vi "Tag_Buffer_Dbl_Input_VIG.vi"(7 "Operation":enum16{"get data", "set data", "initialize"}(ring)=enum."set data", 8 "error in":errorcluster, 9 "Number of Sensors":i32, 11 "tag_data_in":dbl[](array[numeric])) -> (0 "error out":errorcluster, 3 "tag_data_out":dbl[](array[numeric]))   [LabVIEW 2018]
panel:
  # "----TestData Rows---------\n6 -->Flow Rate-(Flow)\n7--->Actual mA (Acutal_Current)\n8-->Temperature (Temp)\n9-->DAQ Sensor 1-Supply Pressure (Supply_Pressure)\n10-->DAQ Sensor 2 - Diff Pressure (50 psid)--(Diff_Pressure_50)\n11-->DAQ Sensor 3 - Back Pressure (output)--(Back_Pressure)\n12-->DAQ Sensor 4- Bypass Pressure--(Bypass_Pressure)\n13-->DAQ Sensor 5 - Diff Pressure (100 psid)--(Diff_Pressure_10)\n14-->DAQ Sensor 6- Unused-(Unused)\n15-->Flow Rate (Raw)--(Flow_Raw)\n16-->Calibrated Flow--(Flow_Cal)\n17-->SG Calibrated --(SG_Cal)"
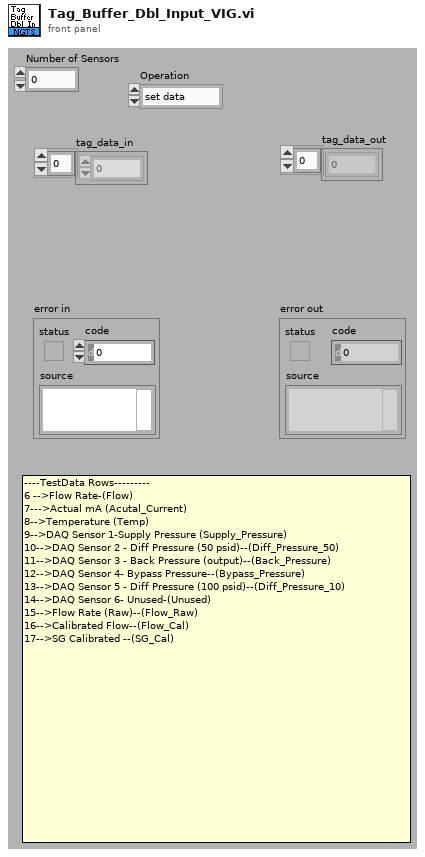
[diagram p1: front panel]
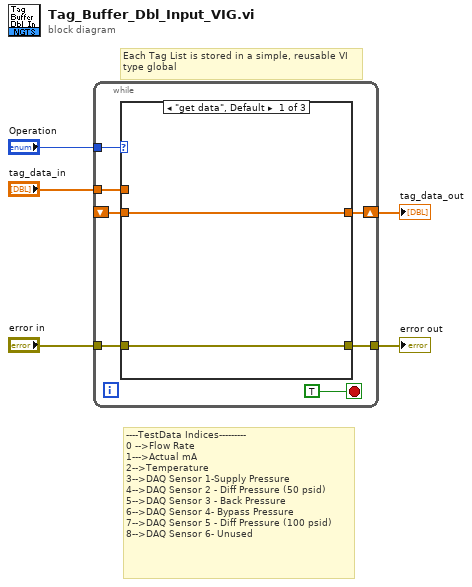
[diagram p0: block diagram]
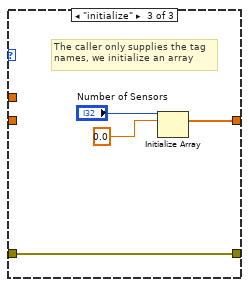
[diagram p3: hidden frame]
diagram:
  # "----TestData Indices---------\n0 -->Flow Rate\n1--->Actual mA \n2-->Temperature\n3-->DAQ Sensor 1-Supply Pressure\n4-->DAQ Sensor 2 - Diff Pressure (50 psid)\n5-->DAQ Sensor 3 - Back Pressure\n6-->DAQ Sensor 4- Bypass Pressure\n7-->DAQ Sensor 5 - Diff Pressure (100 psid)\n8-->DAQ Sensor 6- Unused"
  # "Each Tag List is stored in a simple, reusable VI\ntype global"
  n1 = while {
    tunnel: "Operation" -> [w12]
    shift-right: [w10] -> w3
    shift-left: _ -> [w8]
    tunnel: "tag_data_in" -> [w9]
    tunnel: "error in" -> [w7]
    tunnel: [w6] -> w1
    stop <- TRUE stop-if-true
    n2 = case shown="\"get data\", Default" w12 {
      tunnel: [w14 w16 w20] -> w10
      tunnel: w9 -> [_ w16 _]
      tunnel: w8 -> [w14 _ _]
      tunnel: w7 -> [w13 w15 w19]
      tunnel: [w13 w15 w19] -> w6
      frame "get data", Default {
      }
      frame "set data" {
        # "For speed, we only set the\ndata, not the tag names."
      }
      frame "initialize" {
        # "The caller only supplies the tag\nnames, we initialize an array"
        n3 = Initialize Array(0.0 ("element"), "Number of Sensors") -> (w20:dbl[])
      }
    }
  }
  "error out" <- w1
  "tag_data_out" <- w3
